vi "Zadanie2.vi"() -> ()   [LabVIEW 2011]
panel:
  in  "Numeric 2":dbl
  out "Waveform Chart":dbl(graph)
  out "Numeric":dbl
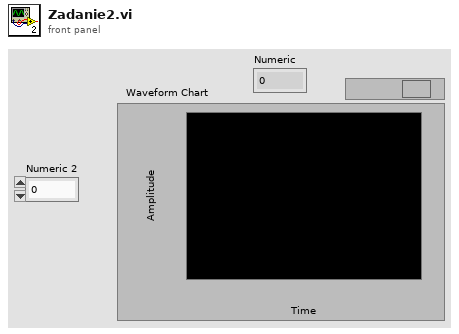
[diagram p1: front panel]
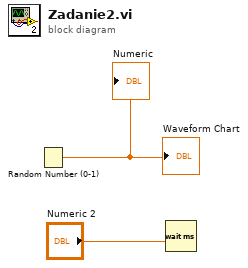
[diagram p0: block diagram]
diagram:
  n1 = Random Number (0-1)() -> (number: 0 to 1=→"Numeric" →"Waveform Chart":dbl)
  n2 = Wait (ms)(milliseconds to wait="Numeric 2") -> ()  [unwired: 1 out]
